vi "Get List Mode.vi"(2 "gen":refnum<class "niUSRP Tx DSP v2 FPGA.lvclass">=refnum) -> (4 "list mode":refnum<class "niVST List Mode Interface v1 FPGA.lvclass">)   [LabVIEW 2023]
uses:
  <instrlib>/niUSRP/Reference FPGA/Tx DSP/niUSRP Tx DSP v2 FPGA.lvclass
  <instrlib>/niVST/List Mode/Interface/v1/FPGA/niVST List Mode Interface v1 FPGA.lvclass
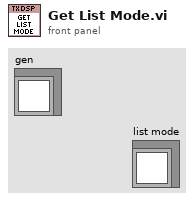
[diagram p1: front panel]
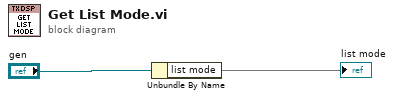
[diagram p0: block diagram]
diagram:
  n1 = Unbundle By Name("gen") -> ("list mode"=→"list mode")
